vi "printlabel.vi"(8 "error in (no error)":errorcluster caption="entrée d'erreur (pas d'erreur)", 10 "para1":string, 11 "para0":string) -> (0 "error out":errorcluster caption="sortie d'erreur", 1 "function return":i32, 2 "para1 out":string, 3 "para0 out":string)   [LabVIEW 2020, in "Library Instrument & Equipement.lvlib" / "Library Printer.lvlib" / "TSCLIB.lvlib"]
doc: "EXPORT int CALLBACK printlabel(char *, char *);"
uses:
  TSCLIB.lvlib
  TSCLIB.dll
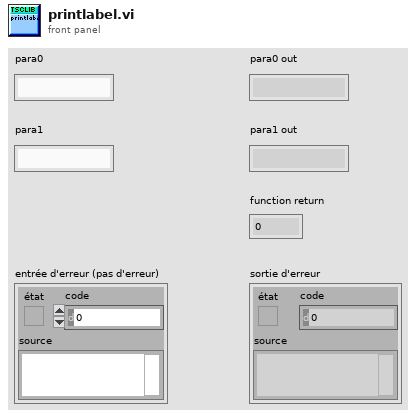
[diagram p1: front panel]
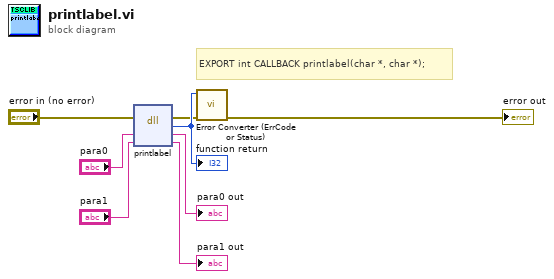
[diagram p0: block diagram]
diagram:
  # "EXPORT int CALLBACK printlabel(char *, char *);"
  n1 = dll-call lib="C:/Users/ngarcin/OneDrive - Altyor/Standard TB/Class/Printer/Printer TSC/TSCLIB/TSCLIB.*" fn="printlabel"(error in="error in (no error)", "para0"="para0", "para1"="para1") -> (error out=w2:errorcluster, w8:i32, "para0"=→"para0 out":string, "para1"=→"para1 out":string)  [unwired: 2 in, 1 out]
  "function return" <- w8
  n2 = call "Error Converter (ErrCode or Status).vi"("error in (no error)"=w2, "error code"=w8) -> ("error out"=→"error out":errorcluster)  [unwired: 9 in]
